vi "Trace Color.vi"(10 "Color":u32, 11 "Cluster in":cluster{"Command":string, "Color":u32}) -> (3 "Cluster out":cluster{"Command":string, "Color":u32})   [LabVIEW 2017]
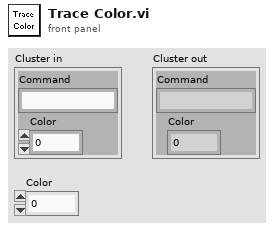
[diagram p1: front panel]
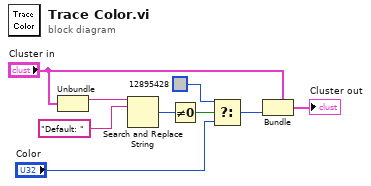
[diagram p0: block diagram]
diagram:
  n1 = Unbundle("Cluster in") -> ("Command"=w7:string)  [unwired: 1 out]
  n2 = Search and Replace String(input string=w7, search string="Default: ") -> (number of replacements=w5:i32)  [unwired: 6 in, 3 out]
  n3 = Not Equal To 0?(x=w5) -> (x != 0?=w4:bool)
  n4 = Select(t=u32 12895428, s=w4, f="Color") -> (s? t:f=w1:u32)
  n5 = Bundle(cluster="Cluster in", "Color"=w1) -> (→"Cluster out":cluster{"Command":string, "Color":u32})  [unwired: 1 in]
